vi "set default gain.vi"(8 "error in (no error)":errorcluster, 11 "Thorcam in":refnum<class "Thorcam.lvclass">) -> (0 "error out":errorcluster, 3 "Thorcam out":refnum<class "Thorcam.lvclass">)   [LabVIEW 2012, in "Thorcam.lvclass"]
uses:
  Thorcam.lvclass
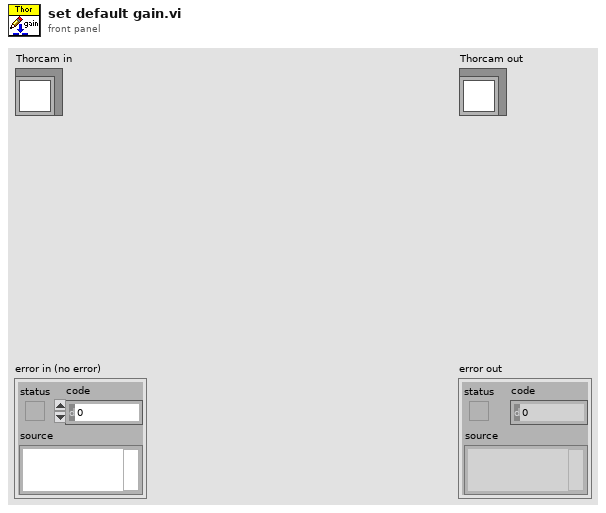
[diagram p1: front panel]
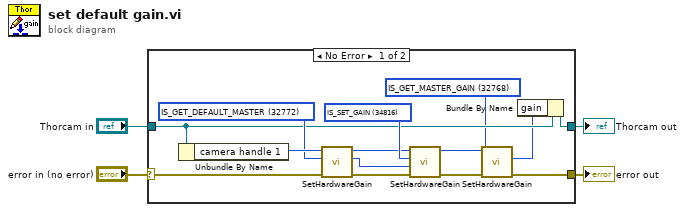
[diagram p0: block diagram]
diagram:
  n1 = case shown="No Error" "error in (no error)" {
    selector: "error in (no error)" -> [w16 w20]
    tunnel: [w8 w20] -> w3
    tunnel: [w10 w19] -> w1
    tunnel: "Thorcam in" -> [w11 w19]
    frame No Error {
      w5 = 32768 items=["IS_GET_MASTER_GAIN"=32768, "IS_GET_RED_GAIN"=32769, "IS_GET_GREEN_GAIN"=32770, "IS_GET_BLUE_GAIN"=32771, "IS_GET_DEFAULT_MASTER"=32772, "IS_GET_DEFAULT_RED"=32773, "IS_GET_DEFAULT_GREEN"=32774, "IS_GET_DEFAULT_BLUE"=32775, "IS_SET_GAIN"=34816] ("Mode")
      w13 = 34816 items=["IS_GET_MASTER_GAIN"=32768, "IS_GET_RED_GAIN"=32769, "IS_GET_GREEN_GAIN"=32770, "IS_GET_BLUE_GAIN"=32771, "IS_GET_DEFAULT_MASTER"=32772, "IS_GET_DEFAULT_RED"=32773, "IS_GET_DEFAULT_GREEN"=32774, "IS_GET_DEFAULT_BLUE"=32775, "IS_SET_GAIN"=34816] ("Mode")
      w17 = 32772 items=["IS_GET_MASTER_GAIN"=32768, "IS_GET_RED_GAIN"=32769, "IS_GET_GREEN_GAIN"=32770, "IS_GET_BLUE_GAIN"=32771, "IS_GET_DEFAULT_MASTER"=32772, "IS_GET_DEFAULT_RED"=32773, "IS_GET_DEFAULT_GREEN"=32774, "IS_GET_DEFAULT_BLUE"=32775, "IS_SET_GAIN"=34816] ("Mode")
      n2 = Unbundle By Name(w11) -> ("camera handle 1"=w18:u32)
      n3 = call <instrlib>:"SetHardwareGain.vi"("error in"=w16, "Mode"=w17, "Camera Handle In"=w18) -> ("error out"=w15:errorcluster, "Value"=w14:i32, "Camera Handle Out"=w12:u32)  [unwired: 6 in]
      n4 = call <instrlib>:"SetHardwareGain.vi"("error in"=w15, "Master Gain"=w14, "Mode"=w13, "Camera Handle In"=w12) -> ("error out"=w9:errorcluster, "Camera Handle Out"=w7:u32)  [unwired: 5 in, 1 out]
      n5 = call <instrlib>:"SetHardwareGain.vi"("error in"=w9, "Mode"=w5, "Camera Handle In"=w7) -> ("error out"=w8:errorcluster, "Value"=w6:i32)  [unwired: 6 in, 1 out]
      n6 = Bundle By Name(cluster=w11, "gain"=w6) -> (w10:refnum<class "Thorcam.lvclass">)
    }
    frame Error {
    }
  }
  "error out" <- w3
  "Thorcam out" <- w1
